vi "9068-Main.vi"(8 "error in (no error)":errorcluster, 9 "run time":u32=60, 10 "target alias":string="cRIO", 11 "configuration file path":path=path "/home/lvuser/RT_Exec_Timing.pcfg") -> (0 "error out":errorcluster)   [LabVIEW 2014]
doc: "This application launches and executes the Tag Bus Data framework configuration for the specified target alias. This is a simple example of the framework API functions, but may also be a suitable starting point for a Host UI or Thick Client that is running a local version of the framework."
uses:
  <vilib>/NI/Module Execution Interface/Engine Runtime/Execution States.ctl
  <vilib>/NI/Module Execution Interface/Engine Runtime/Fault.ctl
  <vilib>/NI/Tag Bus Module Framework/runtime/error classification.ctl
  <vilib>/NI/Module Execution Interface/Engine Runtime/Engine Runtime Interface.lvclass
  <vilib>/NI/DCAF/Tag Editor Core/Framework Configuration Classes/target runtime/PL_Target Runtime.lvclass
  <vilib>/NI/Tag Bus Module Framework/runtime/TBM module execution interface.lvclass
panel:
  out "engine status":T4(array[cluster])
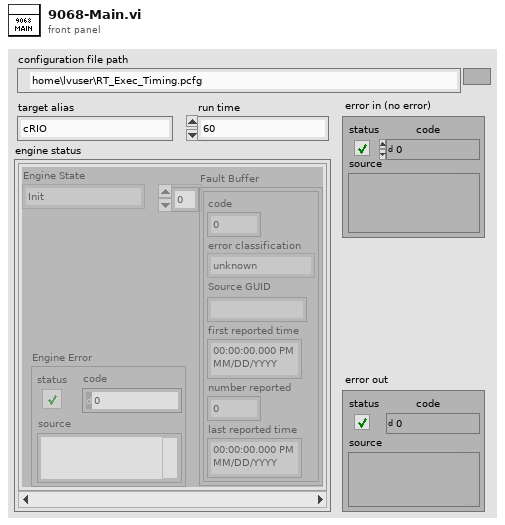
[diagram p1: front panel]
types:
  T1 = typedef "Engine Runtime Interface.lvclass/Execution States.ctl" = enum16{"Init", "Pre-Operational", "Safe-Operational", "Operational", "Stopped"}
  T2 = typedef "Engine Runtime Interface.lvclass/Fault.ctl" = cluster{"code":i32, "error classification":T3, "Source GUID":string, "first reported time":timestamp, "number reported":u32, "last reported time":timestamp}
  T3 = typedef "TBM module execution interface.lvclass/error classification.ctl" = enum16{"unknown", "none", "trivial", "recoverable", "critical"}
  T4 = cluster{"Engine State":T1, "Fault Buffer":T2[], "Engine Error":errorcluster}[]
  T5 = cluster{"Engine State":T1, "faults":T2[], "Engine Error":errorcluster}
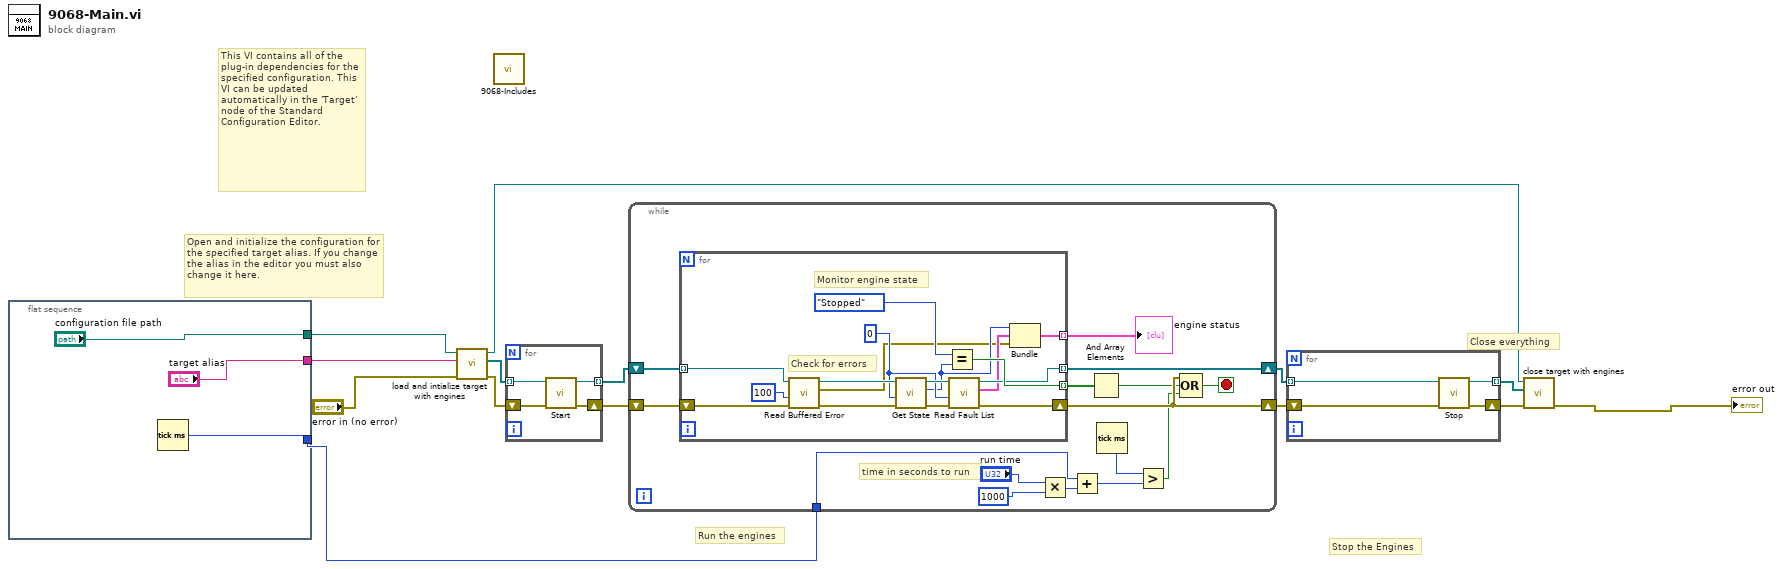
[diagram p0: block diagram]
diagram:
  # "Open and initialize the configuration for the specified target alias. If you change the alias in the editor you must also change it here."
  # "Close everything"
  # "Stop the Engines"
  # "This VI contains all of the plug-in dependencies for the specified configuration. This VI can be updated automatically in the 'Target' node of the Standard Configuration Editor."
  # "Run the engines"
  n1 = flat-sequence {
    tunnel: ["target alias"] -> w9
    tunnel: ["configuration file path"] -> w5
    tunnel: [w15] -> w3
    frame #0 {
      n2 = Tick Count (ms)() -> (millisecond timer value=w15:u32)
    }
  }
  n3 = call <vilib>:"load and intialize target with engines.vi"("error in"="error in (no error)", "target alias"=w9, "file path"=w5) -> ("error out"=w11:errorcluster, "engine runtime interfaces"=w10:refnum<class "Engine Runtime Interface.lvclass">[], "target runtime"=w7:refnum<class "PL_Target Runtime.lvclass">)  [unwired: 6 in]
  n4 = call "9068-Includes.vi"() -> ()  [unwired: 12 in]
  n5 = for {
    tunnel: [w21] -> w14 mode=indexing
    tunnel: w10 -> [w18] mode=indexing
    shift-right: [w20] -> w4
    shift-left: w11 -> [w19]
    n6 = call-dynamic "Start.vi"("error in"=w19, "Engine Runtime Interface in"=w18) -> ("error out"=w20:errorcluster, "Engine Runtime Interface out"=w21:refnum<class "Engine Runtime Interface.lvclass">)  [unwired: 8 in]
  }
  n7 = while {
    shift-right: [w34] -> w13
    shift-left: w14 -> [w36]
    shift-right: [w32] -> w12
    shift-left: w4 -> [w35]
    tunnel: w3 -> [w23]
    stop <- w33 stop-if-true
    # "time in seconds to run"
    n8 = for {
      tunnel: w36 -> [w52] mode=indexing
      tunnel: [w43] -> w34 mode=indexing
      tunnel: [w47] -> w30 mode=indexing
      shift-right: [w42] -> w32
      shift-left: w35 -> [w51]
      tunnel: [w37] -> w31 mode=indexing
      w41 = 0 ("timeout (-1)")
      # "Monitor engine state"
      # "Check for errors"
      n9 = call-dynamic "Read Buffered Error.vi"("error in"=w51, "timeout in ms (0)"=100, "Engine Runtime Interface in"=w52) -> ("error out"=w49:errorcluster, "Engine Error"=w38:errorcluster, "Engine Runtime Interface out"=w50:refnum<class "Engine Runtime Interface.lvclass">)  [unwired: 6 in]
      n10 = call-dynamic "Get State.vi"("error in"=w49, "timeout (-1)"=w41, "Engine Runtime Interface in"=w50) -> ("error out"=w45:errorcluster, "Engine State"=w40:T1, "Engine Runtime Interface out"=w44:refnum<class "Engine Runtime Interface.lvclass">)  [unwired: 6 in]
      n11 = Equal?(x=Execution_States."Stopped" ("Engine State"), y=w40) -> (x = y?=w47:bool)
      n12 = call-dynamic "Read Fault List.vi"("error in"=w45, "timeout (-1)"=w41, "Engine Runtime Interface in"=w44) -> ("error out"=w42:errorcluster, "faults"=w39:T2[], "Engine Runtime Interface out"=w43:refnum<class "Engine Runtime Interface.lvclass">)  [unwired: 6 in]
      n13 = Bundle("Engine State"=w40, "faults"=w39, "Engine Error"=w38) -> (w37:T5)  [unwired: 1 in]
    }
    "engine status" <- w31
    n14 = Multiply(x="run time", y=u32 1000) -> (x*y=w27:u32)
    n15 = Add(x=w23, y=w27) -> (x+y=w26:u32)
    n16 = And Array Elements(Boolean array=w30) -> (logical AND=w29:bool)
    n17 = Tick Count (ms)() -> (millisecond timer value=w25:u32)
    n18 = Greater?(x=w25, y=w26) -> (0:w22:bool)
    n19 = Compound Arithmetic op=OR(w32, w29, w22) -> (w33:bool)
  }
  n20 = for {
    tunnel: w13 -> [w56] mode=indexing
    shift-right: [w53] -> w6
    shift-left: w12 -> [w55]
    tunnel: [w54] -> w8 mode=indexing
    n21 = call-dynamic "Stop.vi"("error in"=w55, "Engine Runtime Interface in"=w56) -> ("error out"=w53:errorcluster, "Engine Runtime Interface out"=w54:refnum<class "Engine Runtime Interface.lvclass">)  [unwired: 8 in]
  }
  n22 = call <vilib>:"close target with engines.vi"("error in"=w6, "Engine Runtime Interfaces"=w8, "Target Runtime"=w7) -> ("error out"=→"error out":errorcluster)  [unwired: 8 in]
